vi "Add Barista.vi"(8 "error in (no error)":errorcluster, 11 "Coffee Shop in":refnum<class "Coffee Shop.lvclass">) -> (0 "error out":errorcluster, 3 "Coffee Shop out":refnum<class "Coffee Shop.lvclass">)   [LabVIEW 2023, in "Coffee Shop.lvlib" / "Coffee Shop.lvclass"]
doc: "Instantiate a new Barista actor"
uses:
  Coffee Shop.lvclass
  c:/dev/_r/4/eng/lv-core/lvpostprocessingd/lv_mc_x86_64/dist_i386/vi.lib/ActorFramework/Actor/Actor.lvclass
  Worker/Barista/Barista.lvclass
  Entity Table/Entity Data.ctl
  Entity Types.ctl
  Coffee Shop.lvclass/Coffee Shop.ctl
  Entity Table/Entity Table.lvclass
  <vilib>/ActorFramework/Actor/Actor.lvclass
panel:
  in  "Waiting":string="Waiting..."
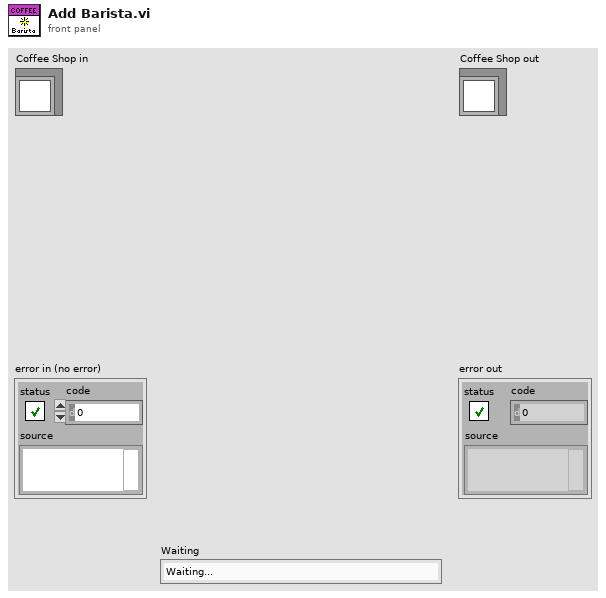
[diagram p1: front panel]
types:
  T1 = typedef "Coffee Shop.lvlib/Coffee Shop.lvclass/Entity Types.ctl" = enum16{"Customer", "Cashier", "Barista"}
  T2 = typedef "Entity Table.lvclass/Entity Data.ctl" = cluster{"Name":string, "Status":string}
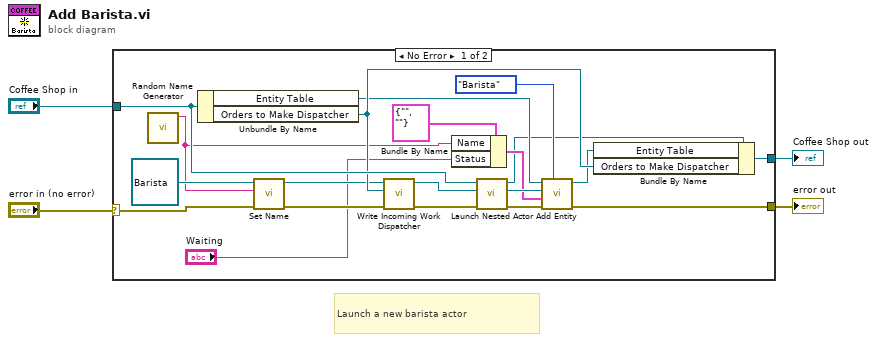
[diagram p0: block diagram]
diagram:
  # "Launch a new barista actor"
  n1 = case shown="No Error" "error in (no error)" {
    selector: "error in (no error)" -> [w24 w26]
    tunnel: [w22 w26] -> w3
    tunnel: [w23 w25] -> w1
    tunnel: "Coffee Shop in" -> [w21 w25]
    frame No Error {
      n2 = call "Random Name Generator.vi"() -> ("Name"=w16:string)  [unwired: 11 in]
      n3 = Unbundle By Name(w21) -> ("Entity Table"=w9:refnum<class "Entity Table.lvclass">, "Orders to Make Dispatcher"=w20:refnum<class "Message Enqueuer.lvclass">)
      n4 = call-dynamic "Set Name.vi"("error in (no error)"=w24, "Name"=w16, "Person in"=refnum<class "Barista.lvclass"> refnum ("Barista.lvclass")) -> ("error out"=w15:errorcluster, "Person out"=w17:refnum<class "Barista.lvclass">)  [unwired: 7 in]
      n5 = call-dynamic "Write Incoming Work Dispatcher.vi"("error in (no error)"=w15, "Incoming Work Dispatcher Queue"=w20, "Worker in"=w17) -> ("error out"=w13:errorcluster, "Worker out"=w6:refnum<class "Barista.lvclass">)  [unwired: 7 in]
      n6 = Bundle By Name(cluster=T2 {"Name"="", "Status"=""} ("Entity"), "Name"=w16, "Status"="Waiting") -> (w10:T2)
      n7 = call <vilib>:"Launch Nested Actor.vi"("error in (no error)"=w13, "Nested Actor"=w6, "Caller Actor in"=w21) -> ("error out"=w12:errorcluster, "Nested Actor's Enqueuer"=w11:refnum<class "Message Enqueuer.lvclass">, "Caller Actor out"=w5:refnum<class "Coffee Shop.lvclass">)  [unwired: 6 in]
      n8 = call "Add Entity.vi"("entity type"=Entity_Types."Barista", "error in (no error)"=w12, "entity details"=w10, "enqueuer"=w11, "Entity Table in"=w9) -> ("error out"=w22:errorcluster, "Entity Table out"=w8:refnum<class "Entity Table.lvclass">)  [unwired: 5 in]
      n9 = Bundle By Name(cluster=w5, "Entity Table"=w8, "Orders to Make Dispatcher"=w20) -> (w23:refnum<class "Coffee Shop.lvclass">)
    }
    frame Error {
    }
  }
  "error out" <- w3
  "Coffee Shop out" <- w1
